vi "React to LV BMS Error.vi"(7 "timeout in ms (-1)":i32=-1, 8 "error in":errorcluster, 10 "Emergency Turn Off Notifier":refnum<notifier>, 11 "CAN Session In":T1=refnum) -> (0 "Exit?":bool=TRUE, 3 "CAN Session Out":T1)   [LabVIEW 2016]
uses:
  Program Files (x86)/National Instruments/LabVIEW 2016/examples/robotics/EPOS2 CANOpen Driver/Low Level VIs/Typedefs/CAN Refnum.ctl
  Program Files (x86)/National Instruments/LabVIEW 2016/examples/robotics/EPOS2 CANOpen Driver/Low Level VIs/Typedefs/CAN Session Pointer.ctl
  Program Files (x86)/National Instruments/LabVIEW 2016/examples/robotics/EPOS2 CANOpen Driver/Low Level VIs/Typedefs/CAN Communication References.ctl
  Program Files (x86)/National Instruments/LabVIEW 2016/examples/robotics/EPOS2 CANOpen Driver/Low Level VIs/Typedefs/kill process notifier array.ctl
  Program Files (x86)/National Instruments/LabVIEW 2016/examples/robotics/EPOS2 CANOpen Driver/Low Level VIs/Typedefs/Write Queue.ctl
  Program Files (x86)/National Instruments/LabVIEW 2016/examples/robotics/EPOS2 CANOpen Driver/Low Level VIs/Typedefs/FPGA CAN Frame Cluster.ctl
  RT/Read single CAN.vi
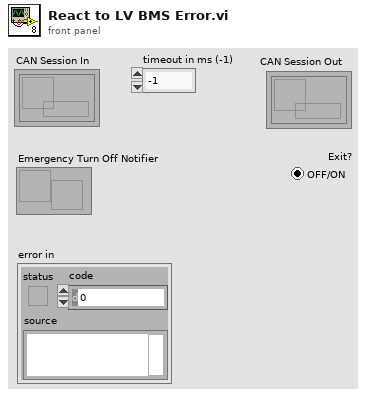
[diagram p1: front panel]
types:
  T1 = typedef "CAN Refnum.ctl" = refnum<k1>
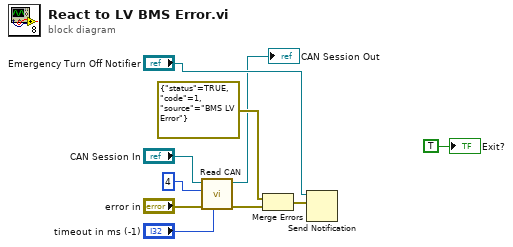
[diagram p0: block diagram]
diagram:
  n1 = call-poly "Read CAN.vi"("timeout in ms (-1)"="timeout in ms (-1)", "error in"="error in", "ID"=4, "CAN Session In"="CAN Session In") -> ("error out"=w9:errorcluster, "CAN Session Out"=→"CAN Session Out":T1)  [unwired: 5 in, 1 out]
  n2 = Merge Errors(errorcluster {"status"=TRUE, "code"=1, "source"="BMS LV Error"} ("error constant"), w9) -> (w8:errorcluster)
  n3 = Send Notification(notification=w8, notifier="Emergency Turn Off Notifier") -> ()  [unwired: 1 in, 2 out]
  "Exit?" <- TRUE
